vi "Stop.vi"(0 "object in":refnum<class "DAQ.lvclass">, 5 "error in (no error)":errorcluster) -> (14 "object out":refnum<class "DAQ.lvclass">, 19 "error out":errorcluster)   [LabVIEW 2021, in "DAQ.lvclass"]
uses:
  DAQ.lvclass
  DAQ.lvclass/DAQ.ctl
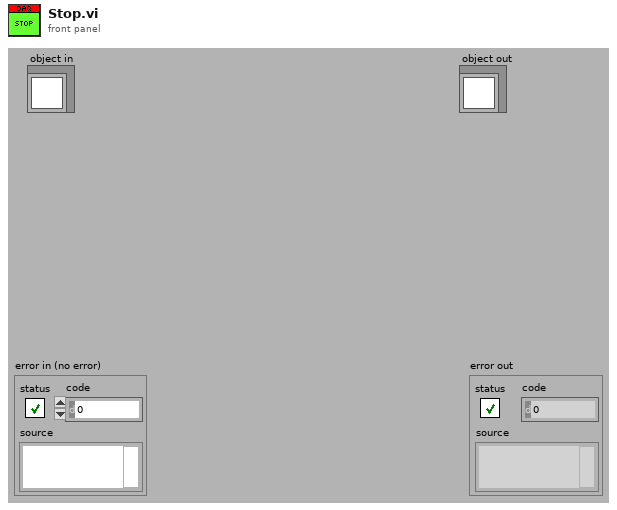
[diagram p1: front panel]
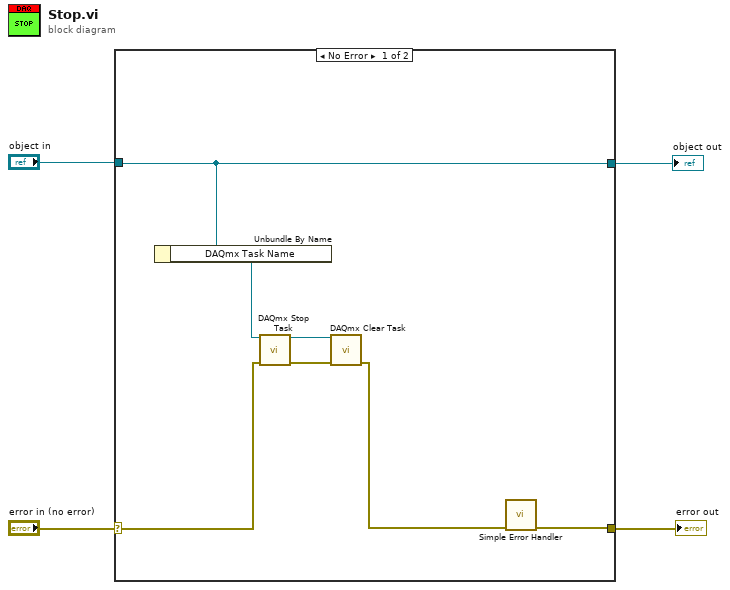
[diagram p0: block diagram]
diagram:
  n1 = case shown="No Error" "error in (no error)" {
    selector: "error in (no error)" -> [w9 w13]
    tunnel: [w6 w13] -> w3
    tunnel: [w5 w12] -> w1
    tunnel: "object in" -> [w5 w12]
    frame No Error {
      n2 = Unbundle By Name(w5) -> ("DAQmx Task Name"=w11:refnum<k21>)
      n3 = call <vilib>:"DAQmx Stop Task.vi"("task/channels in"=w11, "error in"=w9) -> ("task out"=w10:refnum<k21>, "error out"=w8:errorcluster)  [unwired: 12 in]
      n4 = call <vilib>:"DAQmx Clear Task.vi"("task in"=w10, "error in"=w8) -> ("error out"=w7:errorcluster)  [unwired: 13 in]
      n5 = call <vilib>:"Simple Error Handler.vi"("error in (no error)"=w7) -> ("error out"=w6:errorcluster)  [unwired: 4 in, 4 out]
    }
    frame Error {
    }
  }
  "error out" <- w3
  "object out" <- w1
